vi "CastByteArrayAndDispatchMsg.vi"(8 "error in (no error)":errorcluster, 10 "Raw Data":i8[](array[numeric]), 11 "DIMActor in":refnum<class "DIMActor.lvclass">) -> (0 "error out":errorcluster, 3 "DIMActor out":refnum<class "DIMActor.lvclass">)   [LabVIEW 2012, in "DIMActor.lvlib" / "DIMActor.lvclass"]
doc: "Type cast byte array to G data with respect to type descriptor and dispatch message to self.\n\n<b>Needs to be overwitten by derived class.</b>"
uses:
  DIMActor.lvclass
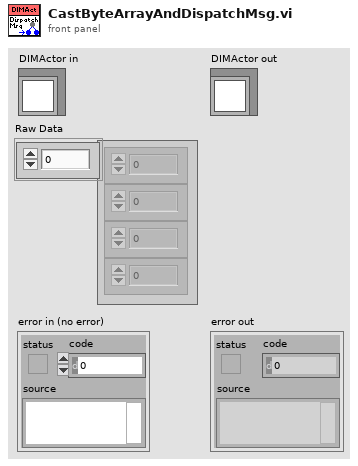
[diagram p1: front panel]
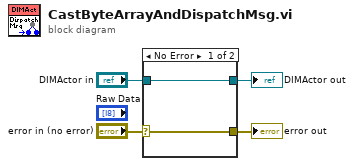
[diagram p0: block diagram]
diagram:
  n1 = case shown="No Error" "error in (no error)" {
    selector: "error in (no error)" -> [w5 w8]
    tunnel: [w5 w8] -> w3
    tunnel: [w6 w7] -> w1
    tunnel: "DIMActor in" -> [w6 w7]
    frame No Error {
    }
    frame Error {
    }
  }
  "error out" <- w3
  "DIMActor out" <- w1
